vi "UFF_Master.vi"(11 "Settings in":T8={"Name of test"="", "Date"=timestamp(0 s since 1904-01-01), "Location"="", "Template"="", "Soundcard"="", "resolution"=32, "Sampling rate"=48000, "Ch1 Gain "=25.0, "Ch2 Gain"=10.0, "Sample time (s)"=0.3, "Pre-trigger (s)"=0.01, "Hammer Threshold"=10.0, "Positions"=12, "Taps/Position"=5, "Set Names"="", "Freq resolution"=10.0, "Hammer cutoff"=0.0, "Mic cutoff"=0.0, "Double bounce "=0.0, "Hammer Cal"=10.0, "dB Offset"=0.0, "Accel Cal"=10.0, "Vibrometer Cal"=0.0, "Mic Cal"=0.0, "Output"=2, "Voltage Cal"=1.0, "Vibrometer Port"="ASRL27::INSTR", "Range"=4, "High Pass"=2, "Bandwidth"=4, "X Range"=[], "Y Range"=[], "dB Spread"=0.0, "Trigger"=0, "Ch_1"=25, "Ch_2"=25, "flip?"=FALSE, "60Hz"=FALSE, "Time offset"=0.0, "Piezo Cal"=1.0, "Default Notes"=""} {"Ch_2" min=1 step=1; "Ch_1" min=1 max=100 step=1; "Trigger" items=["Hammer (force)", "Self-tap", "Spacebar"]; "Bandwidth" items=["1 kHz"=1, "5 kHz"=5, "10 kHz"=10, "25 kHz"=25, "50 kHz"=50, "100 kHz"=100]; "High Pass" items=["Off", "13 Hz", "104 Hz"]; "Range" items=["10 mm/s"=1, "20 mm/s"=2, "50 mm/s"=5, "100 mm/s"=10, "200 mm/s"=20, "500 mm/s"=50, "1 m/s"=100, "2 m/s"=200]; "Output" items=["Accelerometer", "Speed (from acceleration)", "Microphone", "Vibrometer", "Piezo"]; "Voltage Cal" format="%#_13g"; "Ch2 Gain" format="%#_13g"; "Ch1 Gain" format="%#_13g"; "Double bounce" min=0.0; "Mic cutoff" min=0.0 format="%#_4g"; "Hammer cutoff" min=0.0 format="%#_4g"; "Freq resolution" min=0.0; "Pre-trigger (s)" format="%#_13g"; "Date" format="%<%H:%M\n%d/%m/%y>T"; "resolution" items=["16 bit"=16, "24 bit"=24, "32 bit"=32]; "Sampling rate" items=["22050 samp/s"=22050, "44100 samp/s"=44100, "48000 samp/s"=48000]}) -> ()   [LabVIEW 2022 SP3]
uses:
  PreferencesControl.ctl
  <vilib>/Utility/error.llb/Trim Whitespace One-Sided.vi
panel:
  in  "Tab Control":enum32{"Intro", "Params", "Settings", "Saving"}(tab)
  in  "Save Button":bool
  in  "Instrument Name":string(combo)
  in  "Settings":bool
  in  "UFF Path":path
  out "FRF":cluster{"x0":dbl, "df":dbl, dbl[]}[](graph)
  out "Time n Type":T1={"Date"="Frequency", "Time"="Frequency", "Version from DB"=0.0, "Subversion"=0.0, "File Type"=enum."Universal"}
  out "Last Saved":cluster{"Date":string, "Time":string}={"Date"="Frequency", "Time"="Frequency"}
  out "Parent Program":string="Frequency"
  out "Info":T2
  out "Nodes":T3
  out "Units":T4
  out "Conversions":T5
  out "Data":T6(array[cluster]) {"Data"."dX" format="%#.6f"}
  out "transfer fct":cluster{"x0":dbl, "df":dbl, dbl[]}[](graph)
  in  "Back":bool
  out "Tracelines":T7 {"nodes defining" items=["move to node", "draw line to node"]}
  out "Slide":u8(slide) scale=0.0..100.0
  out "Info":string
  # "Welcome To The UFF File Translator"
  # "This will translate a UFF 58 file time (and read the various headers)"
  # "1. Select a file\nHit the folder button or drag a file on"
  # "2. Translate the data\nMake sure the data looks good"
  # "3. Save as an instrument\nAdd to an existing or create a new instrument"
  # "4. Repeat or Close\nOpen a new file or close the window"
  # "Hz"
  # "dB"
  # "dB"
  # "sec"
  # "sec"
  # "mV/Pa"
  # "mV/m/s2"
  # "mV/mm/s"
  # "V/N"
  # "sec"
  # "sec"
  # "mV/N"
  # "a.u."
  # "a.u."
  # "sec"
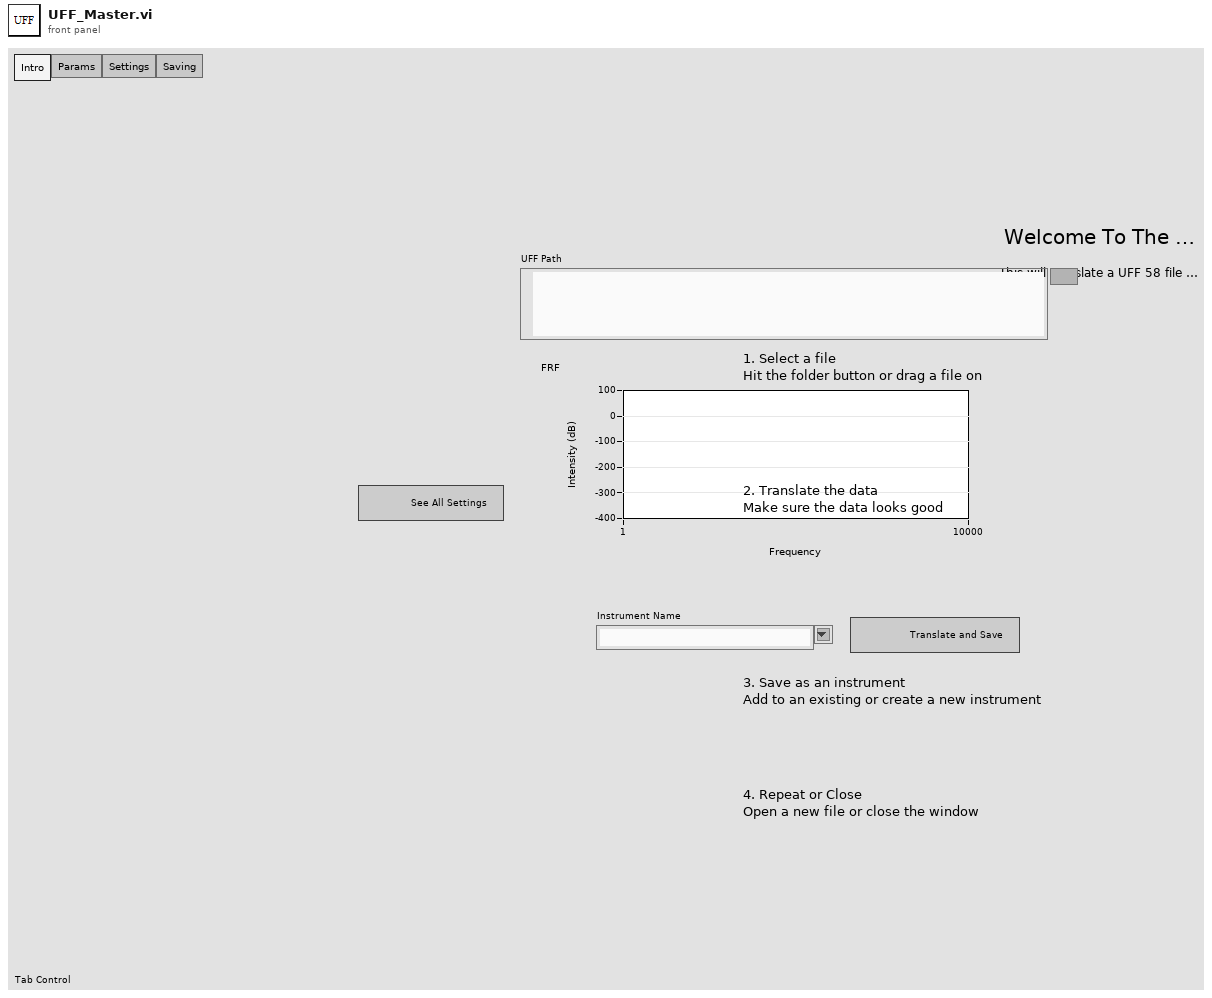
[diagram p1: front panel]
types:
  T1 = cluster{"Date":string, "Time":string, "Version from DB":dbl, "Subversion":dbl, "File Type":enum16{"Universal", "Archive", "Other"}}
  T2 = cluster{"Date file written":string, "Time file written":string, "Release":i32, "Host ID":enum16{"NA", "VAX", "SGI", "HP", "RS", "Alp", "Sun", "Sony", "NEC", "Alop/OSF"}, "Test ID":i32, "Release counter per host":i32}
  T3 = cluster{"Node Label":dbl, "Definition coord sys #":dbl, "Displacement coord sys #":dbl, "Color":dbl, "Coordinates - 1":dbl, "Coordinates - 2":dbl, "Coordinates - 3":dbl}
  T4 = cluster{"Units":enum16{"NA", "SIL: Meter", "BG: Foot", "MG: Meter", "BA: Foot", "MM: millimeter", "CM: cm", "IN: inch", "GM: mm", "US: user defined", "MN: mm"}, "units description":string, "Temperature Mode":enum16{"NA", "absolute", "relaitve"}}
  T5 = cluster{"length conversion":dbl, "force conversion":dbl, "temperature conversion":dbl, "temp offset":dbl}
  T6 = cluster{"Abscissa":cluster{"Specific Data Type":enum16{"Unknown", "general", "stress", "strain", "na1", "temperature", "heat flux", "displacement", "na2", "reaction force", "na3", "velocity", "acceleration", "excitation force", "na4", "pressure", "mass", "time", "frequency", "rpm", "order", "sound pressure", "sound intensity", "sound power"}, "Length unit exponent":i32, "Force units exponent":i32, "Temperature unit exponent":i32, "Axis Label":string, "Axis Label Unit":string}, "Ordinate Numerator":cluster{"Specific Data Type":enum16{"Unknown", "general", "stress", "strain", "na1", "temperature", "heat flux", "displacement", "na2", "reaction force", "na3", "velocity", "acceleration", "excitation force", "na4", "pressure", "mass", "time", "frequency", "rpm", "order", "sound pressure", "sound intensity", "sound power"}, "Length unit exponent":i32, "Force units exponent":i32, "Temperature unit exponent":i32, "Axis Label":string, "Axis Label Unit":string}, "Ordinate Denominator":cluster{"Specific Data Type":enum16{"Unknown", "general", "stress", "strain", "na1", "temperature", "heat flux", "displacement", "na2", "reaction force", "na3", "velocity", "acceleration", "excitation force", "na4", "pressure", "mass", "time", "frequency", "rpm", "order", "sound pressure", "sound intensity", "sound power"}, "Length unit exponent":i32, "Force units exponent":i32, "Temperature unit exponent":i32, "Axis Label":string, "Axis Label Unit":string}, "Z Axis":cluster{"Specific Data Type":enum16{"Unknown", "general", "stress", "strain", "na1", "temperature", "heat flux", "displacement", "na2", "reaction force", "na3", "velocity", "acceleration", "excitation force", "na4", "pressure", "mass", "time", "frequency", "rpm", "order", "sound pressure", "sound intensity", "sound power"}, "Length unit exponent":i32, "Force units exponent":i32, "Temperature unit exponent":i32, "Axis Label":string, "Axis Label Unit":string}, "Data Form":cluster{"Ordinate Data Type":enum16{"NA", "NA2", "Real SGL", "NA3", "Real DBL", "Complex SGL", "Complex DBL"}, "# values or pairs":i32, "Abscissa Spacing":enum16{"Uneven", "Even"}, "Abscissa min":dbl, "Abscissa inc":dbl, "Z Axis Value":dbl}, "DOF ID":cluster{"Function Type":enum16{"General or Unknown", "Time Response", "Auto Spectrum", "Cross Spectrum", "FRF", "Transmissibility", "Coherence", "Auto Correlation", "Cross Correlation", "Power Spectral Density", "Energy Spectral Density Function", "Prob Density Function", "Spectrum", "Cumulative Freq Dist", "Peaks Valley", "Stress/Cycles", "Strain/Cycles", "Orbit", "Mode Indicator Funct", "Force Pattern", "Partial Power", "Partial Coherence", "Eigenvalue", "Eigenvector", "Shock Response Spectrum", "Finite Inpulse Response Filter", "Multiple Coherence", "Order Function", "Phase Compensation"}, "Function ID #":i32, "Version Number":i32, "Load Case ID":enum16{"Single Point Excitation"}, "Response Name":string, "Response Node":i32, "Response Direction":i8, "Reference Name":string, "Reference Node":i32, "Reference Direction":i8}, "Data":cluster{"X0":dbl, "dX":dbl, "Y":dbl[]}, "Header":string}[]
  T7 = cluster{"trace line number":i16, "# nodes defining line":i16, "color":i16, "Identification":string, "nodes defining":u16[]}
  T8 = typedef "PreferencesControl.ctl" = cluster{"Name of test":string, "Date":timestamp, "Location":string, "Template":string, "Soundcard":string, "resolution":u16, "Sampling rate":u16, "Ch1 Gain ":dbl, "Ch2 Gain":dbl, "Sample time (s)":dbl, "Pre-trigger (s)":dbl, "Hammer Threshold":dbl, "Positions":i16, "Taps/Position":i16, "Set Names":string, "Freq resolution":dbl, "Hammer cutoff":dbl, "Mic cutoff":dbl, "Double bounce ":dbl, "Hammer Cal":dbl, "dB Offset":dbl, "Accel Cal":dbl, "Vibrometer Cal":dbl, "Mic Cal":dbl, "Output":u16, "Voltage Cal":dbl, "Vibrometer Port":refnum<visa-resource-name>, "Range":u16, "High Pass":u16, "Bandwidth":u16, "X Range":cluster{"Minimum":dbl, "Maximum":dbl, "Increment":dbl, "Minor Increment":dbl, "Start":dbl}[], "Y Range":cluster{"Minimum":dbl, "Maximum":dbl, "Increment":dbl, "Minor Increment":dbl, "Start":dbl}[], "dB Spread":dbl, "Trigger":u16, "Ch_1":u8, "Ch_2":u8, "flip?":bool, "60Hz":bool, "Time offset":dbl, "Piezo Cal":dbl, "Default Notes":string}
  T9 = cluster{"Abscissa":cluster{"Specific Data Type":enum16{"Unknown", "general", "stress", "strain", "na1", "temperature", "heat flux", "displacement", "na2", "reaction force", "na3", "velocity", "acceleration", "excitation force", "na4", "pressure", "mass", "time", "frequency", "rpm", "order", "sound pressure", "sound intensity", "sound power"}, "Length unit exponent":i32, "Force units exponent":i32, "Temperature unit exponent":i32, "Axis Label":string, "Axis Label Unit":string}, "Ordinate Numerator":cluster{"Specific Data Type":enum16{"Unknown", "general", "stress", "strain", "na1", "temperature", "heat flux", "displacement", "na2", "reaction force", "na3", "velocity", "acceleration", "excitation force", "na4", "pressure", "mass", "time", "frequency", "rpm", "order", "sound pressure", "sound intensity", "sound power"}, "Length unit exponent":i32, "Force units exponent":i32, "Temperature unit exponent":i32, "Axis Label":string, "Axis Label Unit":string}, "Ordinate Denominator":cluster{"Specific Data Type":enum16{"Unknown", "general", "stress", "strain", "na1", "temperature", "heat flux", "displacement", "na2", "reaction force", "na3", "velocity", "acceleration", "excitation force", "na4", "pressure", "mass", "time", "frequency", "rpm", "order", "sound pressure", "sound intensity", "sound power"}, "Length unit exponent":i32, "Force units exponent":i32, "Temperature unit exponent":i32, "Axis Label":string, "Axis Label Unit":string}, "Z Axis":cluster{"Specific Data Type":enum16{"Unknown", "general", "stress", "strain", "na1", "temperature", "heat flux", "displacement", "na2", "reaction force", "na3", "velocity", "acceleration", "excitation force", "na4", "pressure", "mass", "time", "frequency", "rpm", "order", "sound pressure", "sound intensity", "sound power"}, "Length unit exponent":i32, "Force units exponent":i32, "Temperature unit exponent":i32, "Axis Label":string, "Axis Label Unit":string}, "Data Form":cluster{"Ordinate Data Type":enum16{"NA", "NA2", "Real SGL", "NA3", "Real DBL", "Complex SGL", "Complex DBL"}, "# values or pairs":i32, "Abscissa Spacing":enum16{"Uneven", "Even"}, "Abscissa min":dbl, "Abscissa inc":dbl, "Z Axis Value":dbl}, "DOF ID":cluster{"Function Type":enum16{"General or Unknown", "Time Response", "Auto Spectrum", "Cross Spectrum", "FRF", "Transmissibility", "Coherence", "Auto Correlation", "Cross Correlation", "Power Spectral Density", "Energy Spectral Density Function", "Prob Density Function", "Spectrum", "Cumulative Freq Dist", "Peaks Valley", "Stress/Cycles", "Strain/Cycles", "Orbit", "Mode Indicator Funct", "Force Pattern", "Partial Power", "Partial Coherence", "Eigenvalue", "Eigenvector", "Shock Response Spectrum", "Finite Inpulse Response Filter", "Multiple Coherence", "Order Function", "Phase Compensation"}, "Function ID #":i32, "Version Number":i32, "Load Case ID":enum16{"Single Point Excitation"}, "Response Name":string, "Response Node":i32, "Response Direction":i8, "Reference Name":string, "Reference Node":i32, "Reference Direction":i8}, "Data":cluster{dbl, dbl, dbl[]}, "Header":string}[]
  T10 = cluster{"Abscissa":cluster{"Specific Data Type":enum16{"Unknown", "general", "stress", "strain", "na1", "temperature", "heat flux", "displacement", "na2", "reaction force", "na3", "velocity", "acceleration", "excitation force", "na4", "pressure", "mass", "time", "frequency", "rpm", "order", "sound pressure", "sound intensity", "sound power"}, "Length unit exponent":i32, "Force units exponent":i32, "Temperature unit exponent":i32, "Axis Label":string, "Axis Label Unit":string}, "Ordinate Numerator":cluster{"Specific Data Type":enum16{"Unknown", "general", "stress", "strain", "na1", "temperature", "heat flux", "displacement", "na2", "reaction force", "na3", "velocity", "acceleration", "excitation force", "na4", "pressure", "mass", "time", "frequency", "rpm", "order", "sound pressure", "sound intensity", "sound power"}, "Length unit exponent":i32, "Force units exponent":i32, "Temperature unit exponent":i32, "Axis Label":string, "Axis Label Unit":string}, "Ordinate Denominator":cluster{"Specific Data Type":enum16{"Unknown", "general", "stress", "strain", "na1", "temperature", "heat flux", "displacement", "na2", "reaction force", "na3", "velocity", "acceleration", "excitation force", "na4", "pressure", "mass", "time", "frequency", "rpm", "order", "sound pressure", "sound intensity", "sound power"}, "Length unit exponent":i32, "Force units exponent":i32, "Temperature unit exponent":i32, "Axis Label":string, "Axis Label Unit":string}, "Z Axis":cluster{"Specific Data Type":enum16{"Unknown", "general", "stress", "strain", "na1", "temperature", "heat flux", "displacement", "na2", "reaction force", "na3", "velocity", "acceleration", "excitation force", "na4", "pressure", "mass", "time", "frequency", "rpm", "order", "sound pressure", "sound intensity", "sound power"}, "Length unit exponent":i32, "Force units exponent":i32, "Temperature unit exponent":i32, "Axis Label":string, "Axis Label Unit":string}, "Data Form":cluster{"Ordinate Data Type":enum16{"NA", "NA2", "Real SGL", "NA3", "Real DBL", "Complex SGL", "Complex DBL"}, "# values or pairs":i32, "Abscissa Spacing":enum16{"Uneven", "Even"}, "Abscissa min":dbl, "Abscissa inc":dbl, "Z Axis Value":dbl}, "DOF ID":cluster{"Function Type":enum16{"General or Unknown", "Time Response", "Auto Spectrum", "Cross Spectrum", "FRF", "Transmissibility", "Coherence", "Auto Correlation", "Cross Correlation", "Power Spectral Density", "Energy Spectral Density Function", "Prob Density Function", "Spectrum", "Cumulative Freq Dist", "Peaks Valley", "Stress/Cycles", "Strain/Cycles", "Orbit", "Mode Indicator Funct", "Force Pattern", "Partial Power", "Partial Coherence", "Eigenvalue", "Eigenvector", "Shock Response Spectrum", "Finite Inpulse Response Filter", "Multiple Coherence", "Order Function", "Phase Compensation"}, "Function ID #":i32, "Version Number":i32, "Load Case ID":enum16{"Single Point Excitation"}, "Response Name":string, "Response Node":i32, "Response Direction":i8, "Reference Name":string, "Reference Node":i32, "Reference Direction":i8}, "Data":cluster{dbl, dbl, dbl[]}, "Header":string}
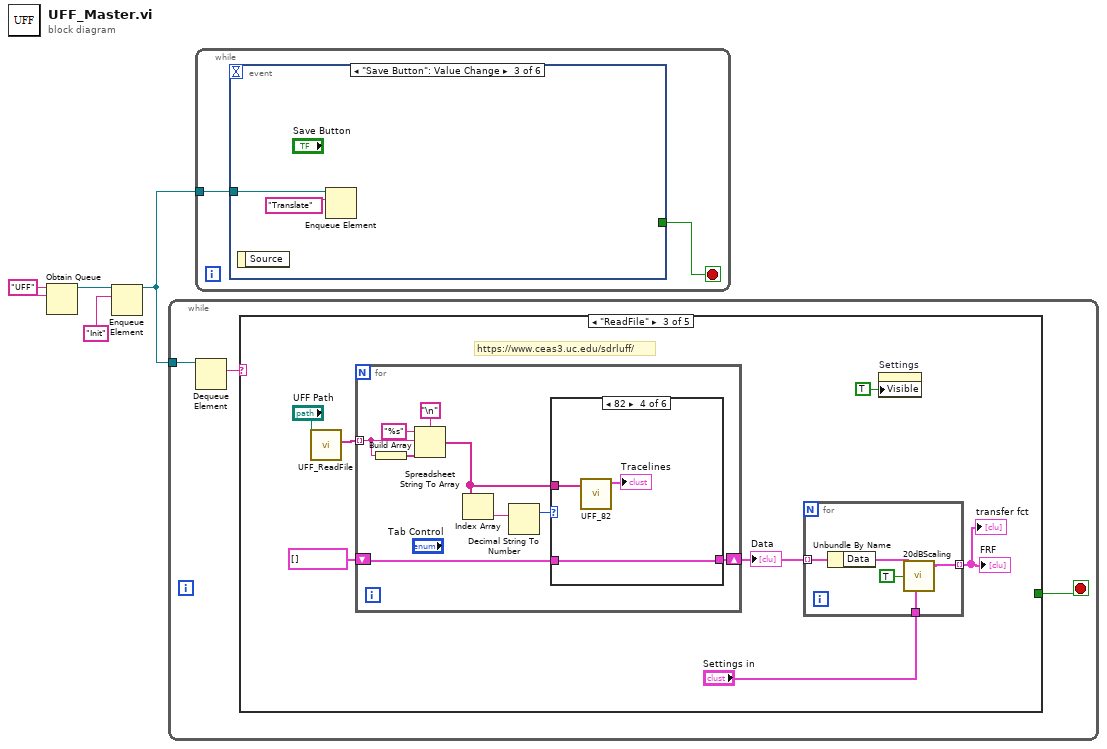
[diagram p0: block diagram]
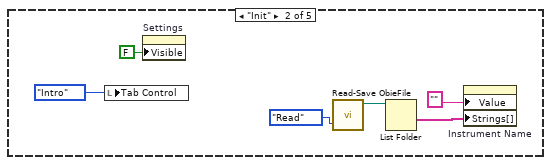
[diagram p3: hidden frame]
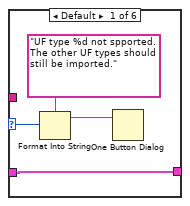
[diagram p4: hidden frame]
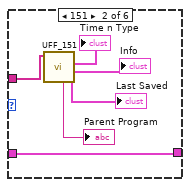
[diagram p5: hidden frame]
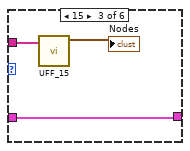
[diagram p6: hidden frame]
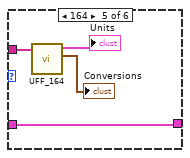
[diagram p7: hidden frame]
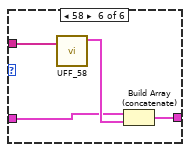
[diagram p8: hidden frame]
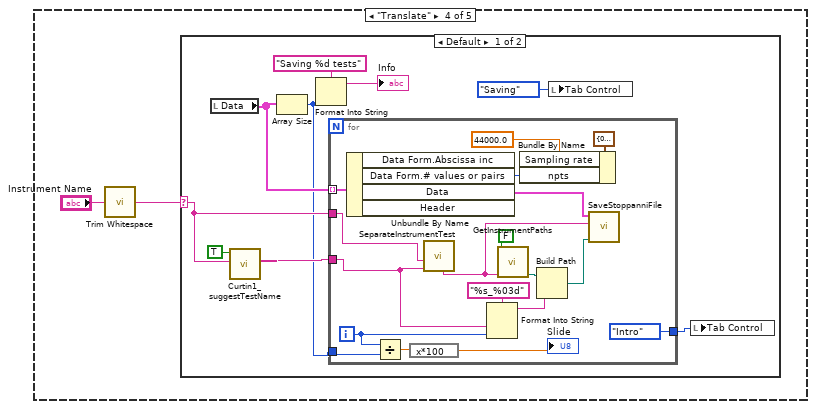
[diagram p9: hidden frame]
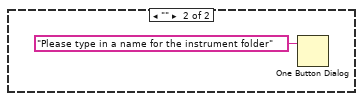
[diagram p10: hidden frame]
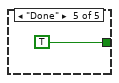
[diagram p11: hidden frame]
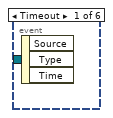
[diagram p12: hidden frame]
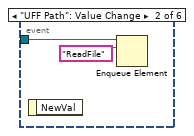
[diagram p13: hidden frame]
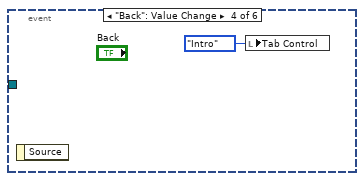
[diagram p14: hidden frame]
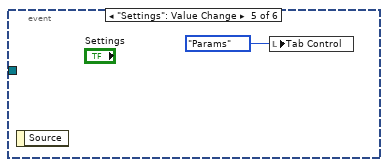
[diagram p15: hidden frame]
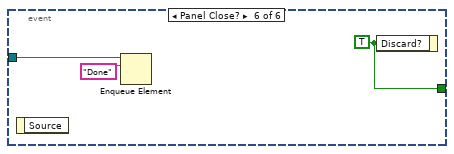
[diagram p16: hidden frame]
diagram:
  w4 = "UFF" ("name (unnamed)")
  n1 = Obtain Queue(name (unnamed)=w4, element data type=w4) -> (queue out=w2:refnum<queue>)  [unwired: 3 in, 2 out]
  n2 = Enqueue Element(queue=w2, element="Init") -> (queue out=w1:refnum<queue>)  [unwired: 2 in, 2 out]
  n3 = while {
    tunnel: w1 -> [w7]
    stop <- w5 stop-if-true
    n4 = Dequeue Element(queue=w7) -> (element=w6:string)  [unwired: 2 in, 3 out]
    n5 = case shown="\"ReadFile\"" w6 {
      tunnel: [_ _ _ _ TRUE ("Discard?")] -> w5
      frame Default {
      }
      frame "Init" {
        n6 = local write "Tab Control"(enum32{"Intro", "Params", "Settings"}."Intro" ("Tab Control")) -> ()
        n7 = property on="Settings" class="Bool"("Visible"=FALSE) -> ()  [unwired: 2 in, 2 out]
        n8 = call "Read-Save ObieFile.vi"("Task"=enum16{"Save", "Read"}."Read") -> ("DataPath Out"=w10:path)  [unwired: 8 in, 2 out]
        n9 = List Folder(path=w10) -> (folder names=w9:string[])  [unwired: 3 in, 3 out]
        n10 = property on="Instrument Name" class="CmbBox"("Value"="" ("Value (Signaling)"), "Strings[]"=w9) -> ()  [unwired: 2 in, 2 out]
      }
      frame "ReadFile" {
        # "https://www.ceas3.uc.edu/sdrluff/"
        n11 = call "UFF_ReadFile.vi"("file (use dialog)"="UFF Path") -> ("packets"=w17:string[])  [unwired: 9 in, 1 out]
        n12 = for {
          tunnel: w17 -> [w31] mode=indexing
          shift-right: [w27] -> w18
          shift-left: T9 [] -> [w26]
          n13 = Build Array(w31) -> (w34:string[])
          n14 = Spreadsheet String To Array(delimiter (Tab)="\n", format string="%s", spreadsheet string=w31, array type (2D Dbl)=w34) -> (array=w29:string[])
          n15 = Index Array(array=w29) -> (element=w28:string)  [unwired: 1 in]
          n16 = Decimal String To Number(string=w28) -> (number=w30:i32)  [unwired: 2 in, 1 out]
          n17 = case shown="82" w30 {
            selector: w30 -> [w37 _ _ _ _ _]
            tunnel: w29 -> [_ w44 w47 w50 w54 w58]
            tunnel: [w38 w39 w45 w49 w51 w56] -> w27
            tunnel: w26 -> [w38 w39 w45 w49 w51 w55]
            frame Default {
              n18 = Format Into String(format string="UF type %d not spported.  The other UF types should still be imported.", w37) -> (resulting string=w35:string)  [unwired: 2 in, 1 out]
              n19 = One Button Dialog(message=w35) -> ()  [unwired: 1 in, 1 out]
            }
            frame 151 {
              n20 = call "UFF_151.vi"("array"=w44) -> ("Last Saved"=→"Last Saved":cluster{"Date":string, "Time":string}, "Info"=→"Info":T2, "Time n Type"=→"Time n Type":T1, "Parent Program"=→"Parent Program":string)  [unwired: 6 in, 1 out]
            }
            frame 15 {
              n21 = call "UFF_15.vi"("array"=w47) -> ("Nodes"=→"Nodes":T3)  [unwired: 10 in]
            }
            frame 82 {
              n22 = call "UFF_82.vi"("array"=w50) -> ("Tracelines"=→"Tracelines":T7)  [unwired: 10 in]
            }
            frame 164 {
              n23 = call "UFF_164.vi"("array"=w54) -> ("Conversions"=→"Conversions":T5, "Units"=→"Units":T4)  [unwired: 9 in]
            }
            frame 58 {
              n24 = call "UFF_58.vi"("array"=w58) -> ("DataSet"=w57:T10)  [unwired: 10 in]
              n25 = Build Array (concatenate)(w55, w57) -> (w56:T9)
            }
          }
        }
        "Data" <- w18
        n26 = for {
          tunnel: w18 -> [w25] mode=indexing
          tunnel: "Settings in" -> [w23]
          tunnel: [w22] -> w14 mode=indexing
          n27 = Unbundle By Name(w25) -> ("Data"=w21:cluster{dbl, dbl, dbl[]})
          n28 = call "20dBScaling.vi"("Average FRF in"=w21, "dB?"=TRUE, "Settings"=w23) -> ("Average FRF out"=w22:cluster{"x0":dbl, "df":dbl, dbl[]})  [unwired: 3 in, 1 out]
        }
        "transfer fct" <- w14
        "FRF" <- w14
        n29 = property on="Settings" class="Bool"("Visible"=TRUE) -> ()  [unwired: 2 in, 2 out]
      }
      frame "Translate" {
        n30 = call <vilib>:"Trim Whitespace.vi"("string"="Instrument Name") -> ("trimmed string"=w59:string)  [unwired: 1 in]
        n31 = case shown="Default" w59 {
          selector: w59 -> [w67 _]
          frame Default {
            n32 = local read "Data"() -> (w68:T6)
            n33 = call "Curtin1_suggestTestName.vi"("instrument"=w67, "Build?"=TRUE) -> ("Suggested Test"=w65:string)  [unwired: 9 in]
            n34 = Array Size(array=w68) -> (size(s)=w63:i32)
            n35 = Format Into String(format string="Saving %d tests", w63) -> (resulting string=→"Info":string)  [unwired: 2 in, 1 out]
            n36 = for {
              tunnel: w68 -> [w87] mode=indexing
              tunnel: w67 -> [w78]
              tunnel: w65 -> [w75]
              tunnel: w63 -> [w73]
              tunnel: [enum32{"Intro", "Params", "Settings", "Saving"}."Intro" ("Tab Control")] -> w61
              i -> [w74]
              n37 = Unbundle By Name(w87) -> ("Data Form.# values or pairs"=w84:i32, "Data"=w82:cluster{"X0":dbl, "dX":dbl, "Y":dbl[]})  [unwired: 2 out]
              n38 = Divide(x=w74, y=w73) -> (x/y=w72:dbl)
              n39 = expression code="x*100"(w72) -> (→"Slide":dbl)
              n40 = call "SeparateInstrumentTest.vi"("test in"=w75, "Instrument in"=w78) -> ("Instrument -- test out"=w81:string)  [unwired: 5 in, 4 out]
              n41 = Format Into String(format string="%s_%03d", w75, w74) -> (resulting string=w76:string)  [unwired: 2 in, 1 out]
              n42 = call "GetInstrumentPaths.vi"("Instrument"=w81, "Build?"=FALSE) -> ("Path To Raw Folder"=w80:path)  [unwired: 5 in, 4 out]
              n43 = Bundle By Name(cluster=cluster{"Sampling rate":dbl, "npts":dbl} {"Sampling rate"=0.0, "npts"=0.0} ("run"), "Sampling rate"=44000.0, "npts"=w84) -> ()  [unwired: 1 out]
              n44 = Build Path(base path=w80, name or relative path=w76) -> (appended path=w79:path)
              n45 = call "SaveStoppanniFile.vi"("Last Path"=w79, "Inst:Test Name"=w81, "Complex FRF"=w82) -> ()  [unwired: 8 in, 1 out]
            }
            n46 = local write "Tab Control"(enum32{"Intro", "Params", "Settings", "Saving"}."Saving" ("Tab Control")) -> ()
            n47 = local write "Tab Control"(w61) -> ()
          }
          frame "" {
            n48 = One Button Dialog(message="Please type in a name for the instrument folder") -> ()  [unwired: 1 in, 1 out]
          }
        }
      }
      frame "Done" {
      }
    }
  }
  n49 = while {
    tunnel: w1 -> [w91]
    stop <- w90 stop-if-true
    n50 = event shown="[2] \"Save Button\": Value Change" {
      selector: _ -> [_ _ _ _ _ _]
      dyn-events: _ -> [_ _ _ _ _ _]
      timeout: _ -> [_ _ _ _ _ _]
      tunnel: w91 -> [_ w93 w95 _ _ w98]
      tunnel: [_ _ _ _ _ w100] -> w90
      event Timeout {
        n51 = event-data() -> ()  [unwired: 1 in, 3 out]
      }
      event "UFF Path": Value Change {
        n52 = event-data() -> ()  [unwired: 1 in, 1 out]
        n53 = Enqueue Element(queue=w93, element="ReadFile") -> ()  [unwired: 2 in, 3 out]
      }
      event "Save Button": Value Change {
        n54 = event-data() -> ()  [unwired: 1 in, 1 out]
        n55 = Enqueue Element(queue=w95, element="Translate") -> ()  [unwired: 2 in, 3 out]
      }
      event "Back": Value Change {
        n56 = event-data() -> ()  [unwired: 1 in, 1 out]
        n57 = local write "Tab Control"(enum32{"Intro", "Params", "Settings"}."Intro" ("Tab Control")) -> ()
      }
      event "Settings": Value Change {
        n58 = event-data() -> ()  [unwired: 1 in, 1 out]
        n59 = local write "Tab Control"(enum32{"Intro", "Params", "Settings"}."Params" ("Tab Control")) -> ()
      }
      event Panel Close? {
        w100 = TRUE ("Discard?")
        n60 = event-data() -> ()  [unwired: 1 in, 1 out]
        n61 = Enqueue Element(queue=w98, element="Done") -> ()  [unwired: 2 in, 3 out]
        n62 = event-data("Discard?"=w100) -> ()  [unwired: 1 in, 1 out]
      }
    }
  }
